vi "Triax320 SetParams.vi"(4 "OutSlit":dbl caption="Output Slit(mm)" format="%#_7g", 5 "CalOffset":i32=-1641 caption="Cal Offset", 6 "InSlit":dbl caption="Input Slit(mm)" format="%#_7g", 7 "Grating Description":string="400nm", 8 "error in":errorcluster, 9 "LineDensity":u32=1800 caption="Line Density\n(Groove/mm)", 10 "Grating":u8(ring) items=["1", "2", "3"], 11 "Param":T1=enum."Tous") -> (0 "error out":errorcluster)   [LabVIEW 2019]
doc: "Ce Vi enregistre les paramètres des différents axes dans un fichier .ini"
uses:
  <userlib>/Triax320/TriaxParams.ctl
  <vilib>/Utility/config.llb/Write Key (U32).vi
  <vilib>/Utility/config.llb/Write Key (Double).vi
  <vilib>/Utility/config.llb/Write Key (String).vi
  <vilib>/Utility/config.llb/Write Key (I32).vi
  <vilib>/Utility/config.llb/NI_LVConfig.lvlib
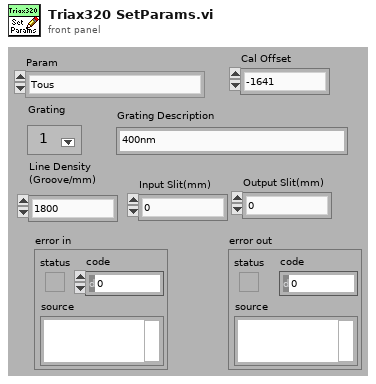
[diagram p1: front panel]
types:
  T1 = typedef "TriaxParams.ctl" = enum16{"Grating", "CalOffset", "Line Density (grv/mm)", "Input Slit (mm)", "Output Slit (mm)", "Both Slit (mm)", "Grating Desc.", "Wavelenght Correction", "Tous"}
  T2 = typedef "NI_LVConfig.lvlib/Config Data RefNum.ctl" = refnum<k1>
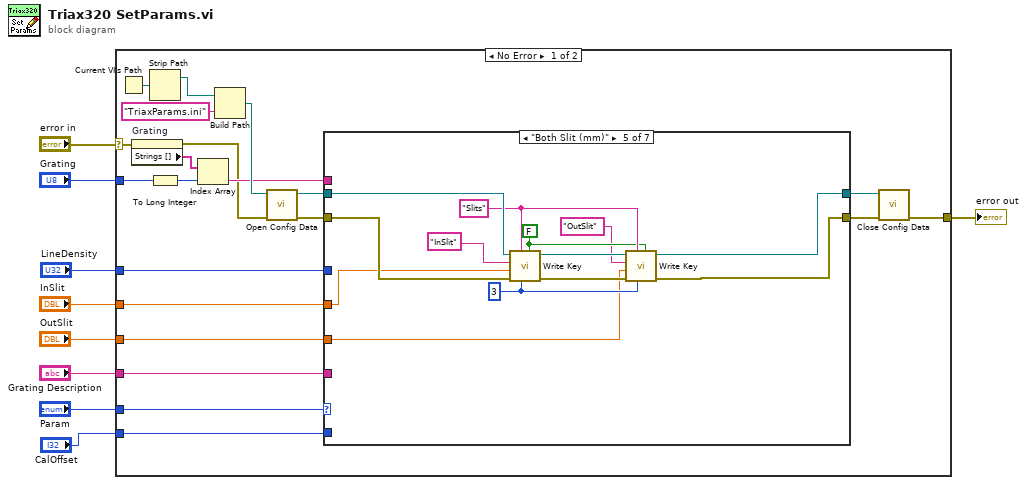
[diagram p0: block diagram]
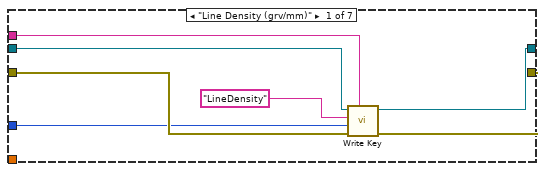
[diagram p2: hidden frame]
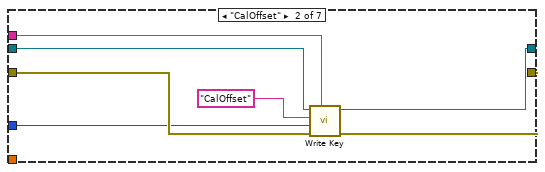
[diagram p3: hidden frame]
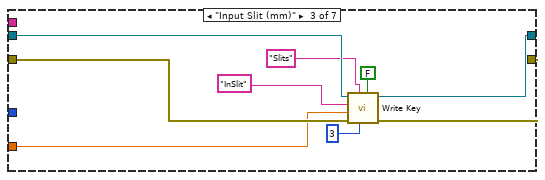
[diagram p4: hidden frame]
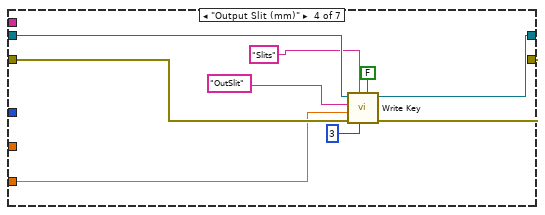
[diagram p5: hidden frame]
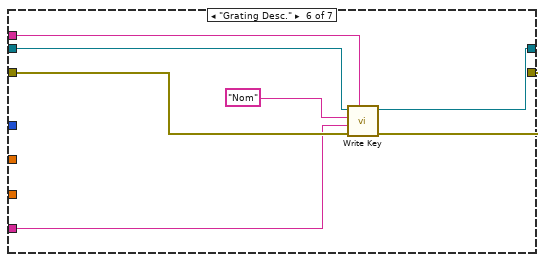
[diagram p6: hidden frame]
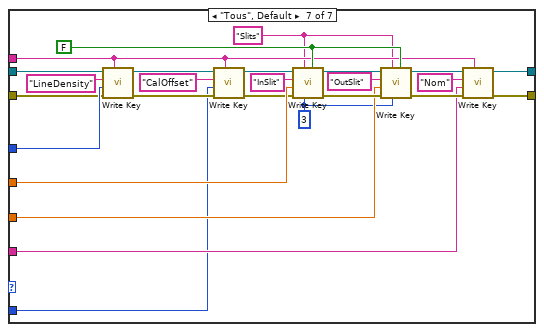
[diagram p7: hidden frame]
diagram:
  n1 = case shown="No Error" "error in" {
    selector: "error in" -> [w17 w109]
    tunnel: "Grating" -> [w27 _]
    tunnel: [w23 w109] -> w8
    tunnel: "Param" -> [w19 _]
    tunnel: "Grating Description" -> [w15 _]
    tunnel: "OutSlit" -> [w14 _]
    tunnel: "LineDensity" -> [w13 _]
    tunnel: "InSlit" -> [w11 _]
    tunnel: "CalOffset" -> [w10 _]
    frame No Error {
      n2 = Current VI's Path() -> (path=w30:path)
      n3 = property on="Grating" class="Ring (strict)"(error in=w17) -> (error out=w16:errorcluster, "Strings []"=w26:string[])  [unwired: 1 in, 1 out]
      n4 = Strip Path(path=w30) -> (stripped path=w18:path)  [unwired: 1 out]
      n5 = To Long Integer(number=w27) -> (32bit integer=w12:i32)
      n6 = Index Array(array=w26, index=w12) -> (element=w22:string)
      n7 = Build Path(base path=w18, name or relative path="TriaxParams.ini") -> (appended path=w28:path)
      n8 = call <vilib>:"Open Config Data.vi"("error in (no error)"=w16, "configuration file path"=w28) -> ("error out"=w24:errorcluster, "refnum"=w25:T2)  [unwired: 7 in, 1 out]
      n9 = case shown="\"Both Slit (mm)\"" w19 {
        tunnel: w25 -> [w34 w41 w51 w60 w75 w79 w92]
        tunnel: w24 -> [w33 w40 w50 w59 w74 w78 w91]
        tunnel: w22 -> [w37 w44 _ _ _ w82 w84]
        tunnel: [w36 w43 w53 w62 w68 w81 w93] -> w21
        tunnel: [w35 w42 w52 w61 w70 w80 w94] -> w20
        tunnel: w15 -> [_ _ _ _ _ w77 w95]
        tunnel: w14 -> [_ _ _ w55 w64 _ w100]
        tunnel: w13 -> [w32 w39 _ _ _ _ w99]
        tunnel: w11 -> [_ _ w48 _ w63 _ w98]
        tunnel: w10 -> [_ _ _ _ _ _ w88]
        frame "Line Density (grv/mm)" {
          n10 = call-poly <vilib>:"Write Key.vi"("section"=w37, "error in (no error)"=w33, "value"=w32, "key"="LineDensity", "refnum"=w34) -> ("error out"=w36:errorcluster, "refnum out"=w35:T2)  [unwired: 4 in, 1 out]
        }
        frame "CalOffset" {
          n11 = call-poly <vilib>:"Write Key.vi"("section"=w44, "error in (no error)"=w40, "value"=w39, "key"="CalOffset", "refnum"=w41) -> ("error out"=w43:errorcluster, "refnum out"=w42:T2)  [unwired: 4 in, 1 out]
        }
        frame "Input Slit (mm)" {
          n12 = call-poly <vilib>:"Write Key.vi"("use system decimal point (T)"=FALSE, "precision (6)"=i16 3, "section"="Slits", "error in (no error)"=w50, "value"=w48, "key"="InSlit", "refnum"=w51) -> ("error out"=w53:errorcluster, "refnum out"=w52:T2)  [unwired: 2 in, 1 out]
        }
        frame "Output Slit (mm)" {
          n13 = call-poly <vilib>:"Write Key.vi"("use system decimal point (T)"=FALSE, "precision (6)"=i16 3, "section"="Slits", "error in (no error)"=w59, "value"=w55, "key"="OutSlit", "refnum"=w60) -> ("error out"=w62:errorcluster, "refnum out"=w61:T2)  [unwired: 2 in, 1 out]
        }
        frame "Both Slit (mm)" {
          w67 = "Slits" ("section")
          w72 = i16 3 ("precision (6)")
          w66 = FALSE ("use system decimal point (T)")
          n14 = call-poly <vilib>:"Write Key.vi"("use system decimal point (T)"=w66, "precision (6)"=w72, "section"=w67, "error in (no error)"=w74, "value"=w63, "key"="InSlit", "refnum"=w75) -> ("error out"=w71:errorcluster, "refnum out"=w69:T2)  [unwired: 2 in, 1 out]
          n15 = call-poly <vilib>:"Write Key.vi"("use system decimal point (T)"=w66, "precision (6)"=w72, "section"=w67, "error in (no error)"=w71, "value"=w64, "key"="OutSlit", "refnum"=w69) -> ("error out"=w68:errorcluster, "refnum out"=w70:T2)  [unwired: 2 in, 1 out]
        }
        frame "Grating Desc." {
          n16 = call-poly <vilib>:"Write Key.vi"("section"=w82, "error in (no error)"=w78, "value"=w77, "key"="Nom", "refnum"=w79) -> ("error out"=w81:errorcluster, "refnum out"=w80:T2)  [unwired: 4 in, 1 out]
        }
        frame "Tous", Default {
          w83 = "Slits" ("section")
          w97 = FALSE ("use system decimal point (T)")
          w96 = i16 3 ("precision (6)")
          n17 = call-poly <vilib>:"Write Key.vi"("section"=w84, "error in (no error)"=w91, "value"=w99, "key"="LineDensity", "refnum"=w92) -> ("error out"=w90:errorcluster, "refnum out"=w89:T2)  [unwired: 4 in, 1 out]
          n18 = call-poly <vilib>:"Write Key.vi"("section"=w84, "error in (no error)"=w90, "value"=w88, "key"="CalOffset", "refnum"=w89) -> ("error out"=w86:errorcluster, "refnum out"=w85:T2)  [unwired: 4 in, 1 out]
          n19 = call-poly <vilib>:"Write Key.vi"("use system decimal point (T)"=w97, "precision (6)"=w96, "section"=w83, "error in (no error)"=w86, "value"=w98, "key"="InSlit", "refnum"=w85) -> ("error out"=w104:errorcluster, "refnum out"=w101:T2)  [unwired: 2 in, 1 out]
          n20 = call-poly <vilib>:"Write Key.vi"("use system decimal point (T)"=w97, "precision (6)"=w96, "section"=w83, "error in (no error)"=w104, "value"=w100, "key"="OutSlit", "refnum"=w101) -> ("error out"=w103:errorcluster, "refnum out"=w102:T2)  [unwired: 2 in, 1 out]
          n21 = call-poly <vilib>:"Write Key.vi"("section"=w84, "error in (no error)"=w103, "value"=w95, "key"="Nom", "refnum"=w102) -> ("error out"=w93:errorcluster, "refnum out"=w94:T2)  [unwired: 4 in, 1 out]
        }
      }
      n22 = call <vilib>:"Close Config Data.vi"("error in (no error)"=w21, "refnum"=w20) -> ("error out"=w23:errorcluster)  [unwired: 8 in, 1 out]
    }
    frame Error {
    }
  }
  "error out" <- w8
